vi "massajVoltageSimple.vi"() -> ()   [LabVIEW 2021]
uses:
  PicoMoLV/Global Variablesyes.vi
  C:/Program Files/New Focus/New Focus Picomotor Application/Samples/LabVIEW/Model 8742/LabVIEW 2009/CmdLib.dll
panel:
  out "Message":string
  in  "SetZero":bool
  in  "Set Velocity":dbl(slide)=10.0 min=10.0 max=4000.0 step=10.0 scale=0.0..2500.0
  out "FContact":bool caption="END CONTACT"
  in  "Volt Stop F":bool
  in  "Tab Control":enum32{"Coupler", "Feelers"}(tab)
  in  "Coupler On":bool
  out "Volt Plot C":dynamicdata(graph)
  out "Volt Plot F":dynamicdata(graph)
  in  "Feelers On":bool
  in  "Couple B":bool
  out "Direction":dbl
  in  "RIGHT":bool
  in  "LEFT":bool
  in  "Decouple":bool
  in  "LEFT/RIGHT COUPLE":bool
  out "CContact":bool caption="IN CONTACT"
  in  "Volt Stop C":bool
  in  "STOP LOOP 2":bool
  in  "Stop":bool
  out "error out":errorcluster
  out "In Motion":bool
  out "Status:":string
  out "Current Position:":string
  in  "Go":bool
  in  "Relative Move:":string
  in  "Selected Motor:":string(combo)
  in  "Selected Controller:":string(combo)
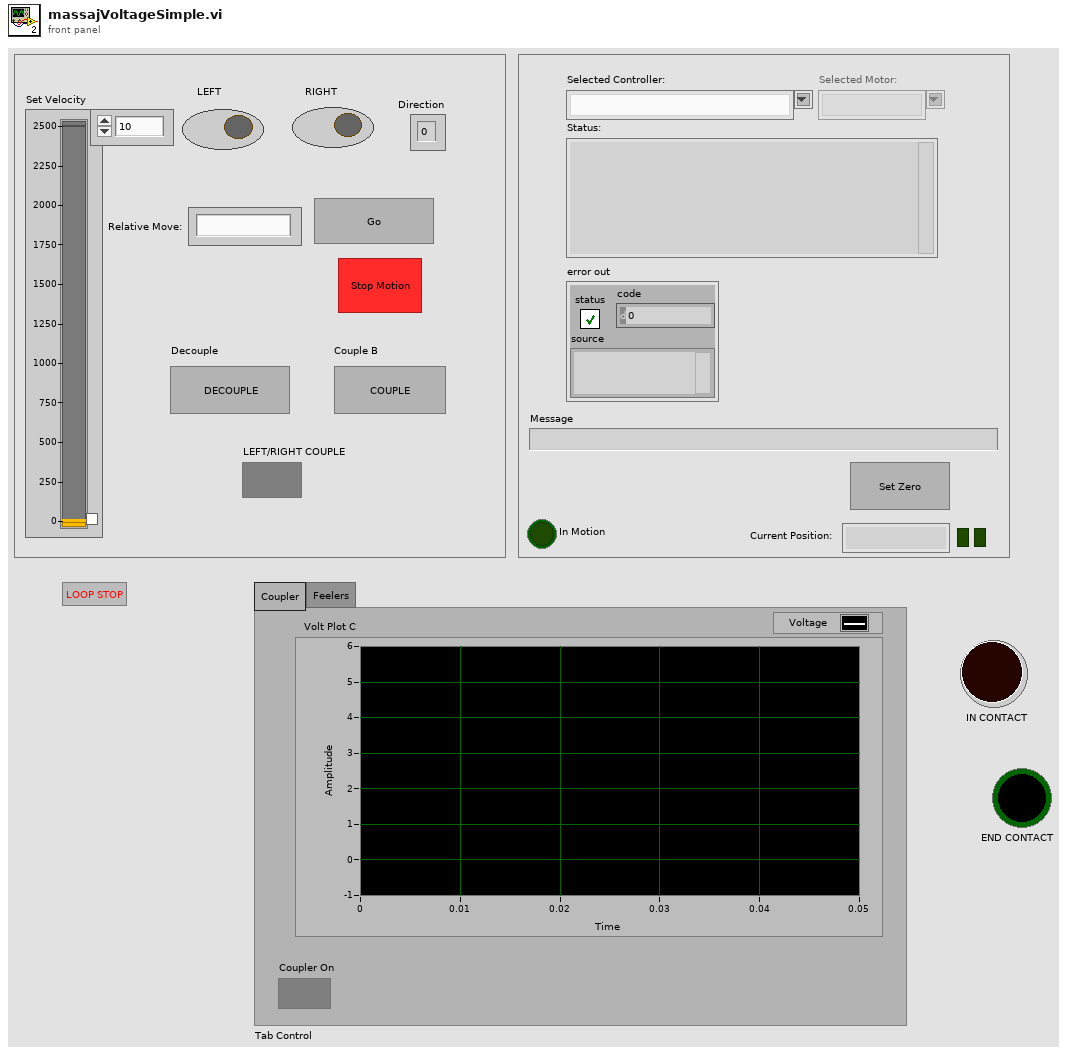
[diagram p1: front panel]
types:
  T1 = cluster{"Selected Controller:":refnum<vi>, "Selected Motor:":refnum<vi>, "Relative Move:":refnum<vi>, "Current Position:":refnum<vi>, "Go":refnum<vi>, "Stop":refnum<vi>}
  T2 = cluster{"DeviceKey":string, "Device Address":i32, "Controller Name":string}[]
  T3 = cluster{"DeviceKey":string, "Device Address":i32, "Controller Name":string}
  T4 = enum8{"Enabled", "Disabled", "Disabled and Grayed Out"}
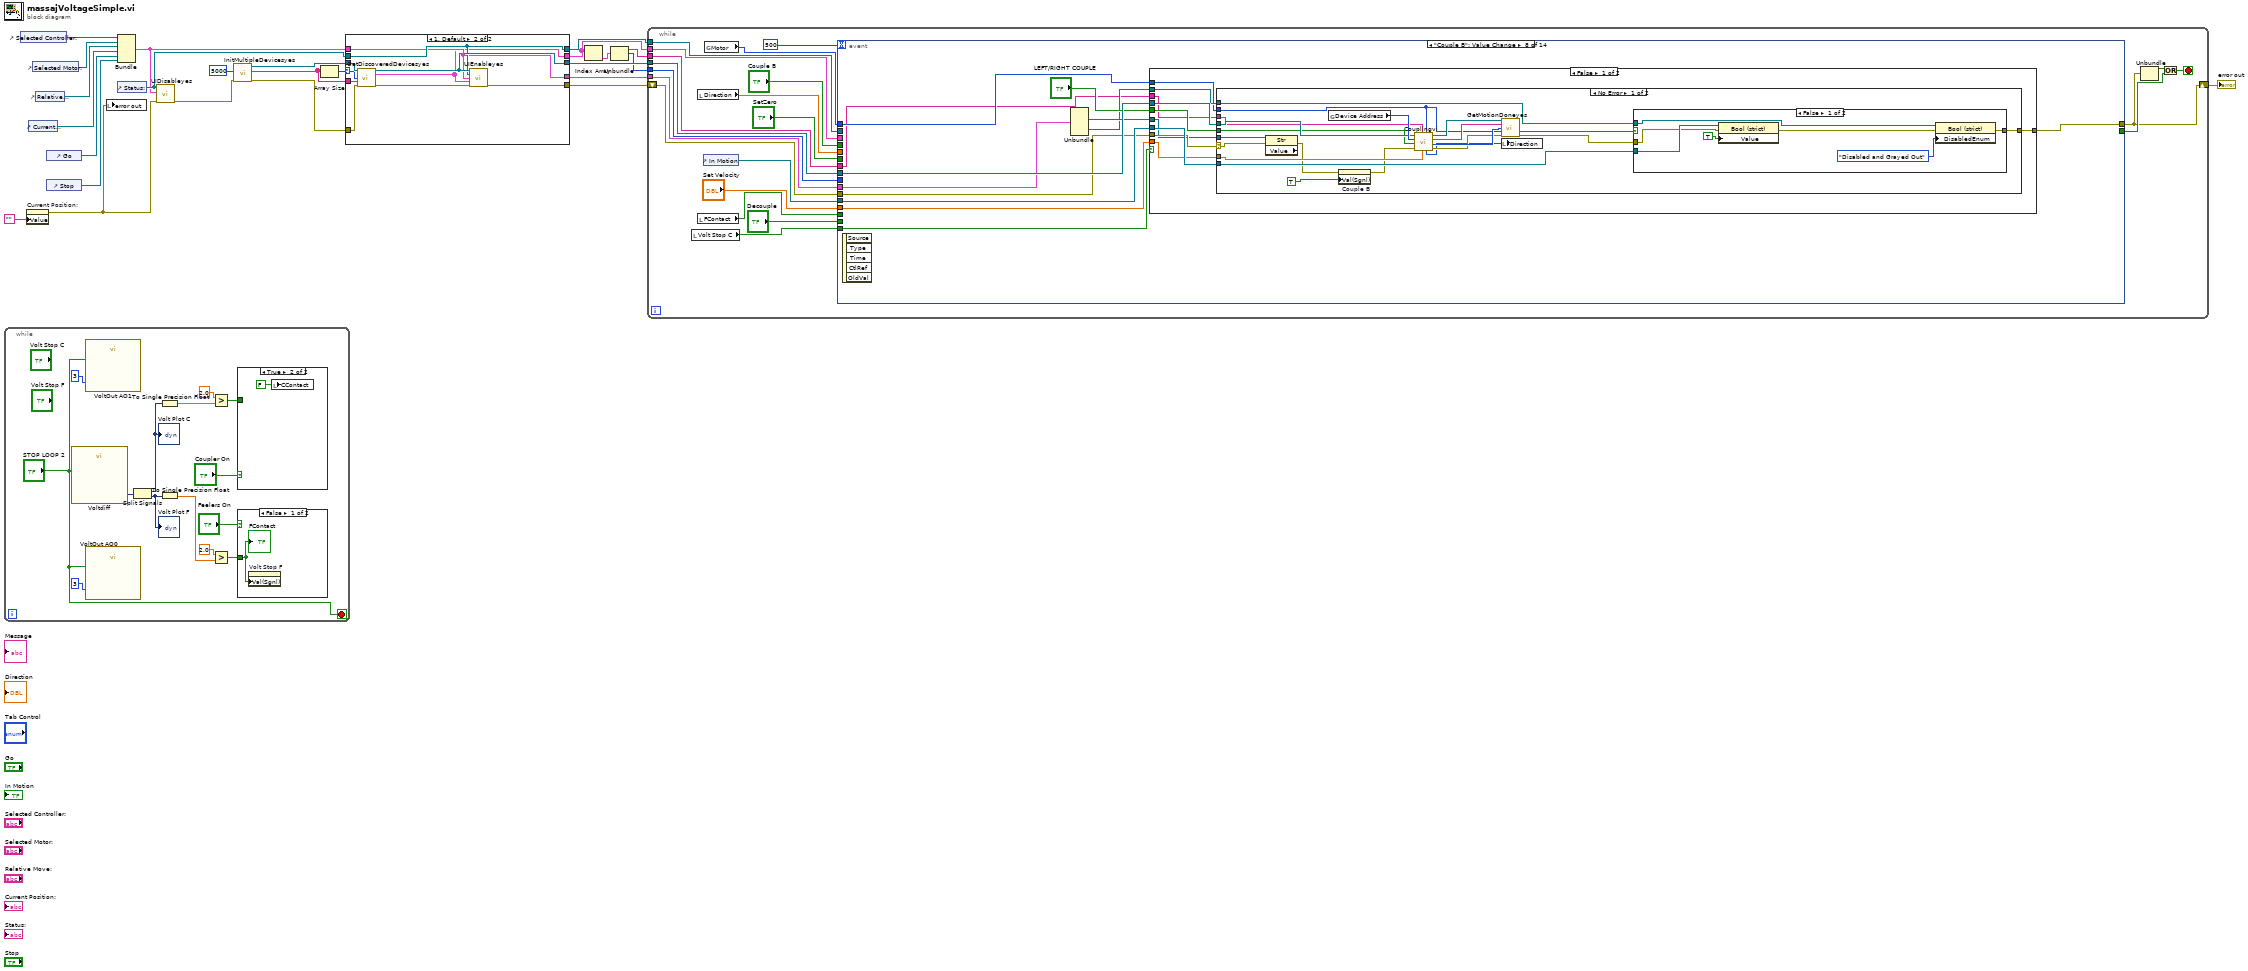
[diagram p0: block diagram]
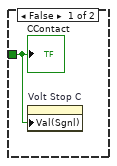
[diagram p2: hidden frame]
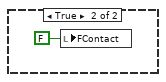
[diagram p3: hidden frame]
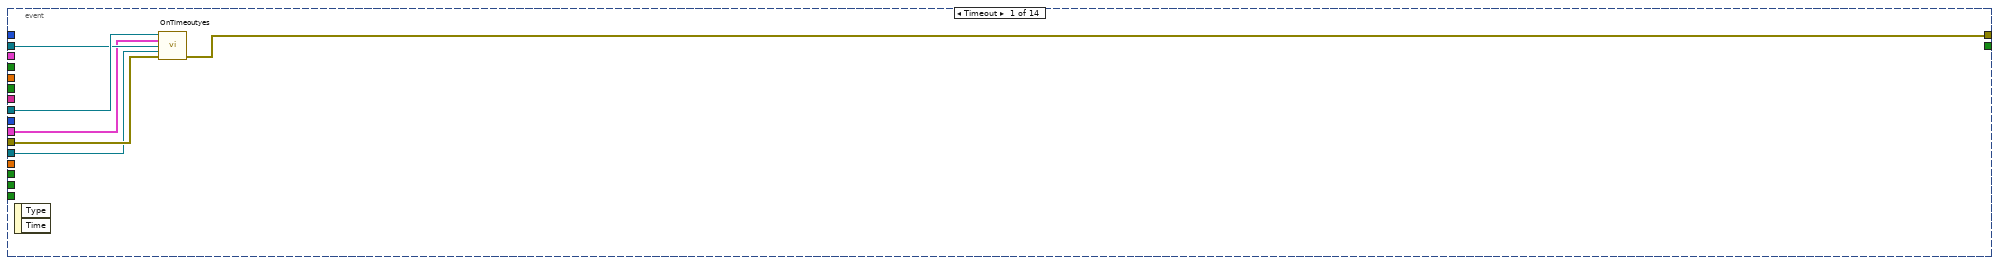
[diagram p4: hidden frame]
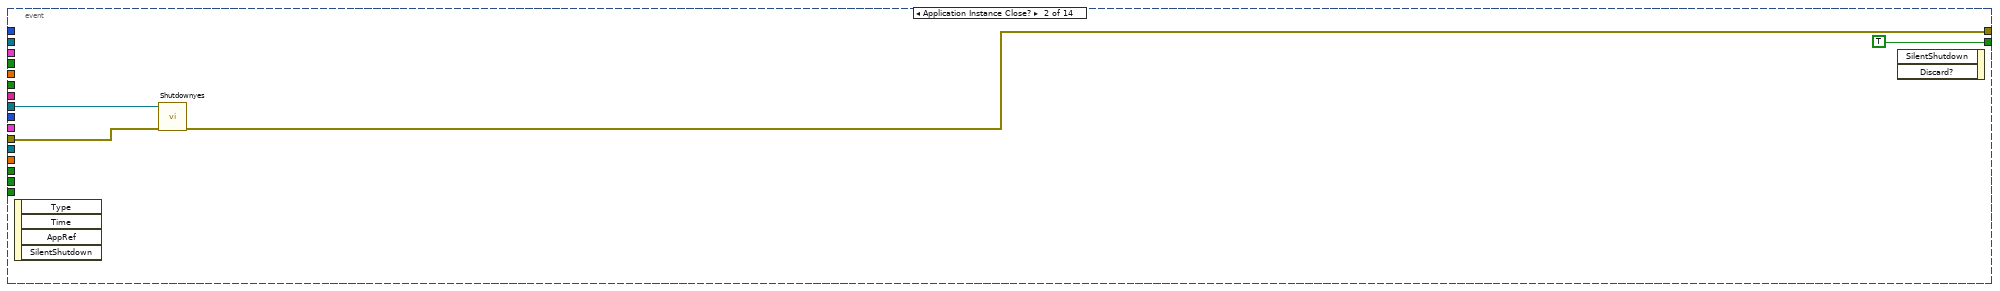
[diagram p5: hidden frame]
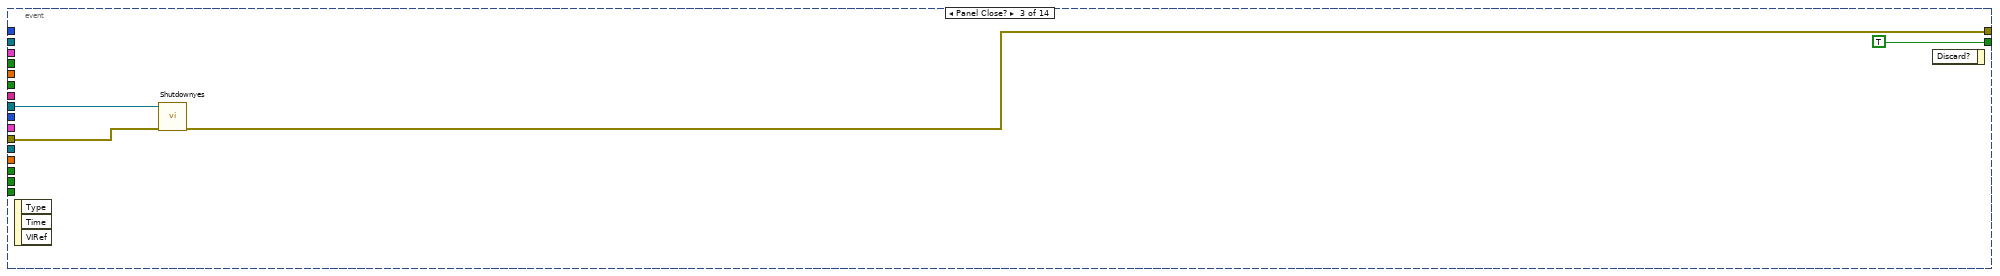
[diagram p6: hidden frame]
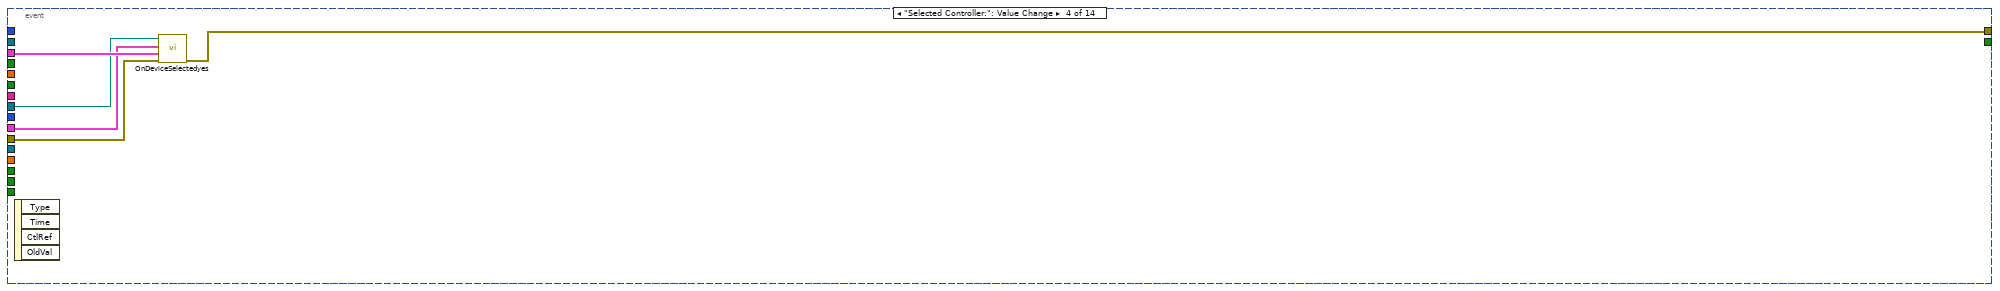
[diagram p7: hidden frame]
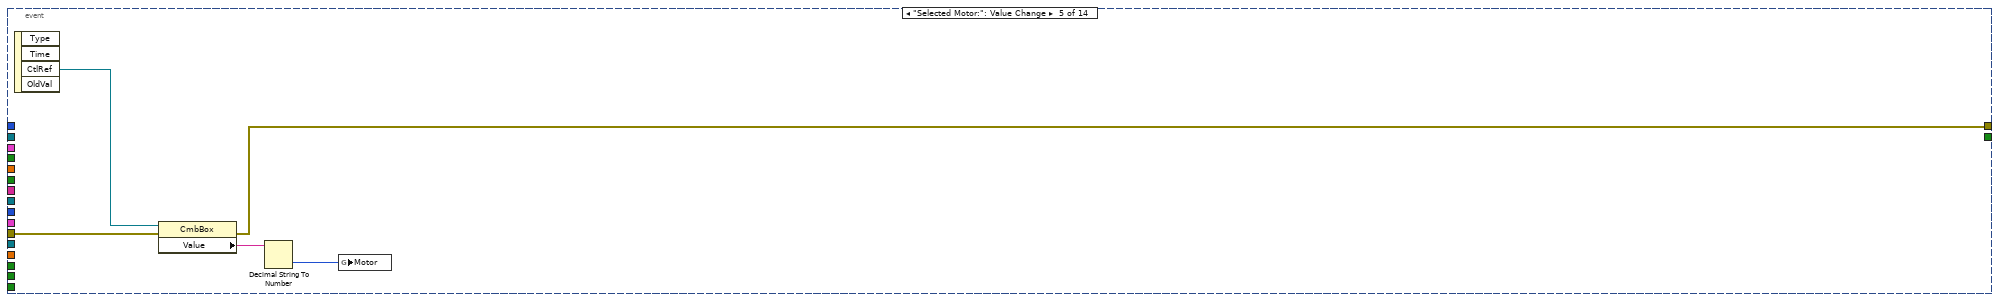
[diagram p8: hidden frame]
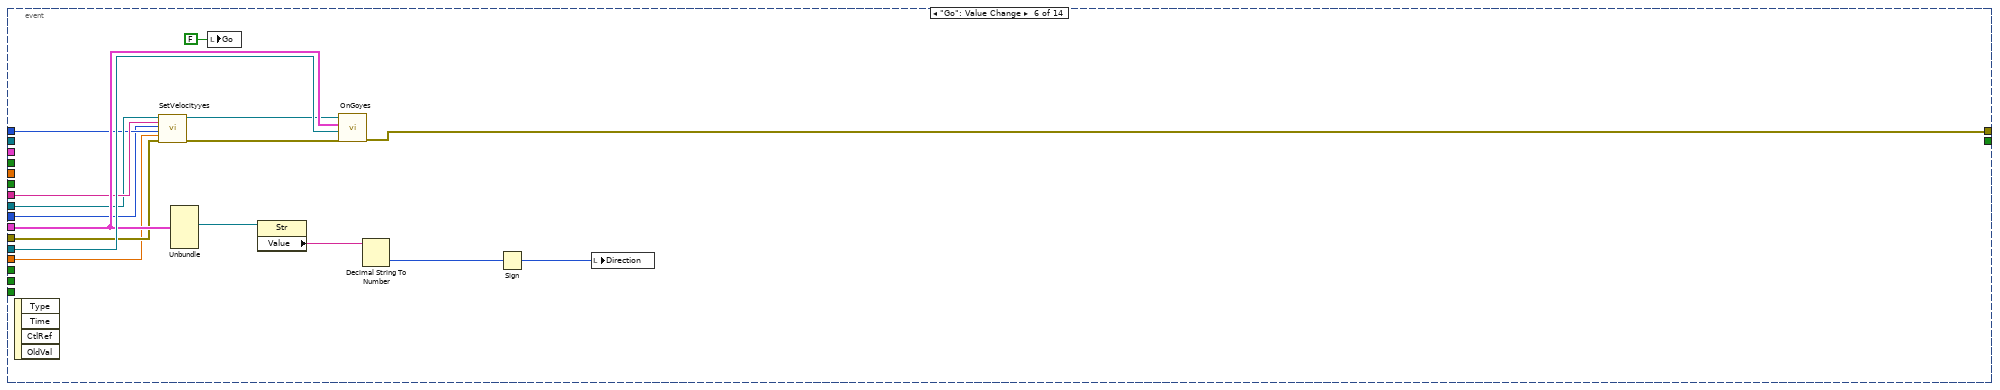
[diagram p9: hidden frame]
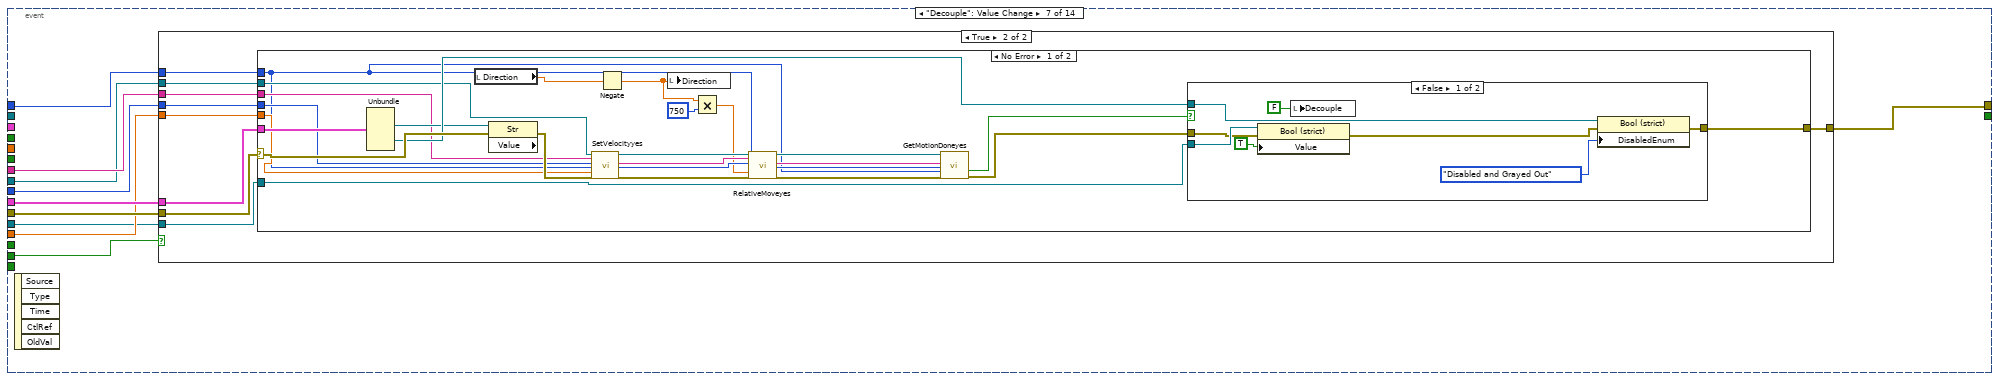
[diagram p10: hidden frame]
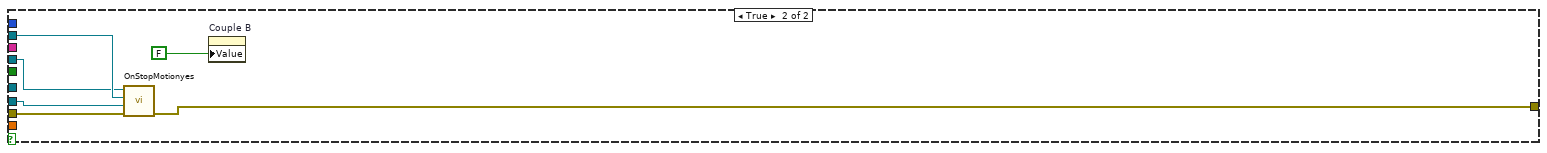
[diagram p16: hidden frame]
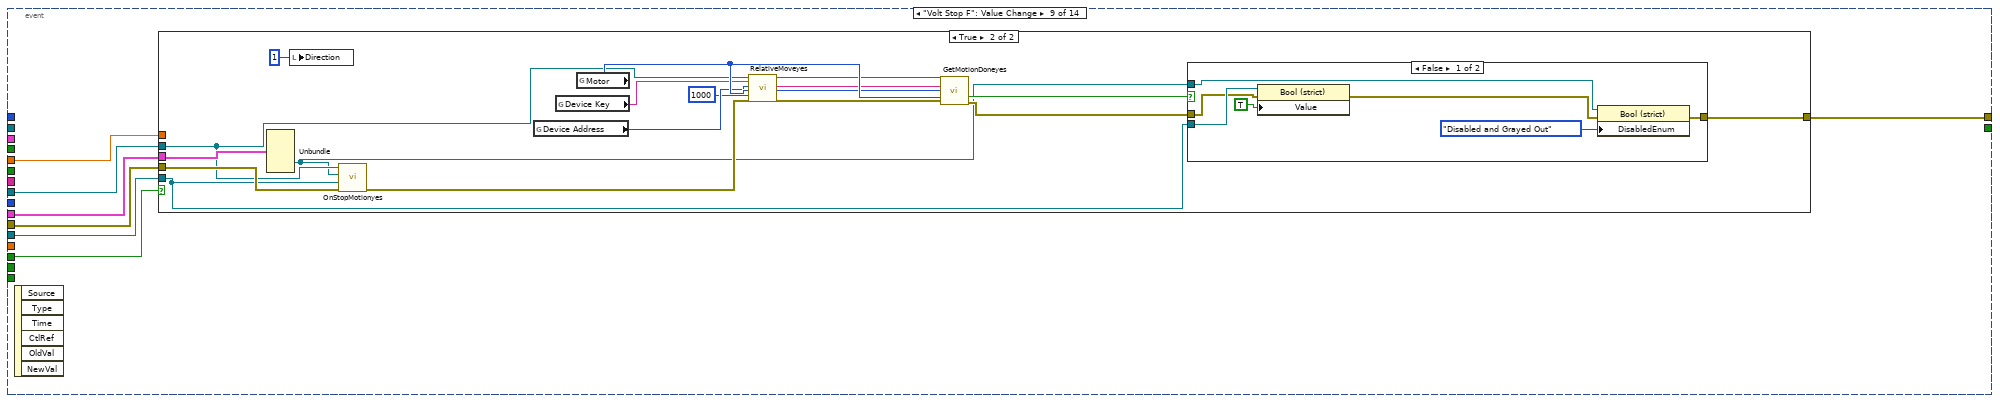
[diagram p17: hidden frame]
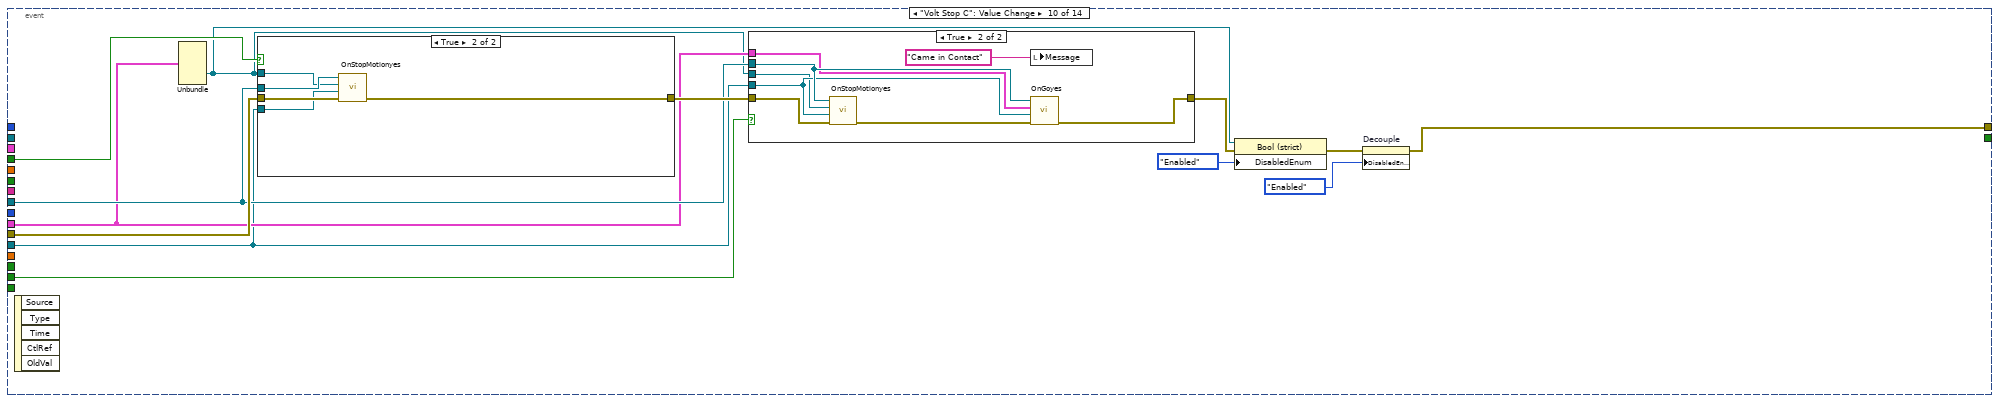
[diagram p20: hidden frame]
diagram:
  n1 = while {
    stop <- "STOP LOOP 2" stop-if-true
    n2 = call "Voltdiff"("stop (F)"="STOP LOOP 2") -> ("data"=w33:dynamicdata)  [unwired: 15 in, 3 out]
    n3 = call "VoltOut AO1"("data"=3, "stop (T)"="STOP LOOP 2") -> ()  [unwired: 16 in, 2 out]
    n4 = call "VoltOut AO0"("data"=3, "stop (T)"="STOP LOOP 2") -> ()  [unwired: 16 in, 2 out]
    n5 = Split Signals(w33) -> (w32:dynamicdata, w28:dynamicdata)  [unwired: 2 in]
    "Volt Plot C" <- w32
    "Volt Plot F" <- w28
    n6 = To Single Precision Float(number=w32) -> (single precision float=w37:sgl)
    n7 = To Single Precision Float(number=w28) -> (single precision float=w30:sgl)
    n8 = Greater?(x=2.0, y=w37) -> (0:w36:bool)
    n9 = Greater?(x=2.0, y=w30) -> (0:w29:bool)
    n10 = case shown="True" "Coupler On" {
      tunnel: w36 -> [w40 _]
      frame False {
        n11 = property on="Volt Stop C" class="Bool (strict)"("Val(Sgnl)"=w40) -> ()  [unwired: 2 in, 2 out]
        "CContact" <- w40
      }
      frame True {
        n12 = local write "CContact"(FALSE) -> ()
      }
    }
    n13 = case shown="False" "Feelers On" {
      tunnel: w29 -> [w42 _]
      frame False {
        n14 = property on="Volt Stop F" class="Bool (strict)"("Val(Sgnl)"=w42) -> ()  [unwired: 2 in, 2 out]
        "FContact" <- w42
      }
      frame True {
        n15 = local write "FContact"(FALSE) -> ()
      }
    }
  }
  n16 = control-ref of="Selected Controller:"() -> (w17:refnum<vi>)
  n17 = property on="Current Position:" class="Str"("Value"="") -> (error out=w8:errorcluster)  [unwired: 2 in, 1 out]
  n18 = control-ref of="Current Position:"() -> (w10:refnum<vi>)
  n19 = control-ref of="Selected Motor:"() -> (w25:refnum<vi>)
  n20 = control-ref of="Relative Move:"() -> (w24:refnum<vi>)
  n21 = control-ref of="Go"() -> (w6:refnum<vi>)
  n22 = control-ref of="Stop"() -> (w7:refnum<vi>)
  n23 = local write "error out"(w8) -> ()
  n24 = Bundle("Selected Controller:"=w17, "Selected Motor:"=w25, "Relative Move:"=w24, "Current Position:"=w10, "Go"=w6, "Stop"=w7) -> (w12:T1)  [unwired: 1 in]
  n25 = control-ref of="Status:"() -> (w16:refnum<vi>)
  n26 = call "UIDisableyes.vi"("error in (no error)"=w8, "UI"=w12, "Status:"=w16) -> ("error out"=w23:errorcluster)  [unwired: 8 in]
  n27 = call "InitMultipleDevicesyes.vi"("error in (no error)"=w23, "msecDelayForDiscovery"=5000) -> ("error out"=w20:errorcluster, "DeviceKey List Out"=w18:string[], "CmdLib Out"=w19:refnum<k24>)  [unwired: 3 in]
  n28 = Array Size(array=w18) -> (size(s)=w21:i32)
  n29 = case shown="1, Default" w21 {
    selector: w21 -> [_ w56]
    tunnel: w16 -> [w45 w53]
    tunnel: w20 -> [w49 w59]
    tunnel: w19 -> [w47 w60]
    tunnel: w18 -> [_ w58]
    tunnel: [w48 w55] -> w15
    tunnel: [w47 w54] -> w14
    tunnel: w12 -> [w46 w52]
    tunnel: [w46 w52] -> w11
    tunnel: [T2 [] ("Device Array") w51] -> w1
    tunnel: [w45 w53] -> w9
    frame 0 {
      n30 = call "AppendToOutputyes.vi"("error in"=w49, "Input String"="No devices were discovered.", "Output Refnum In"=w45) -> ("error out"=w48:errorcluster)  [unwired: 1 in, 1 out]
    }
    frame 1, Default {
      n31 = call "GetDiscoveredDevicesyes.vi"("CmdLib In"=w60, "Master Count"=w56, "DeviceKey List"=w58, "error in"=w59) -> ("CmdLib Out"=w54:refnum<k24>, "Device Array"=w51:T2, "error out"=w57:errorcluster)  [unwired: 9 in]
      n32 = call "UIEnableyes.vi"("CmdLib In"=w54, "Status:"=w53, "UI"=w52, "Device Array"=w51, "error in"=w57) -> ("error out"=w55:errorcluster)  [unwired: 10 in]
    }
  }
  n33 = Index Array(array=w1) -> (element=w4:T3)  [unwired: 1 in]
  n34 = Unbundle(w4) -> ("DeviceKey"=w3:string, "Device Address"=w2:i32)  [unwired: 1 out]
  n35 = while {
    tunnel: w14 -> [w80]
    tunnel: w11 -> [w79]
    tunnel: w1 -> [w78]
    shift-right: [w72] -> w5
    shift-left: w15 -> [w81]
    tunnel: w9 -> [w76]
    tunnel: w3 -> [w64]
    tunnel: w2 -> [w63]
    stop <- w71 stop-if-true
    n36 = local read "Volt Stop C"() -> (w68:bool)
    n37 = local read "Direction"() -> (w66:dbl)
    n38 = local read "FContact"() -> (w67:bool)
    n39 = control-ref of="In Motion"() -> (w73:refnum<vi>)
    n40 = global read "Global Variablesyes.vi" "Motor"() -> (w62:i32)
    n41 = event shown="[7] \"Couple B\": Value Change" {
      selector: _ -> [_ _ _ _ _ _ _ _ _ _ _ _ _ _]
      dyn-events: _ -> [_ _ _ _ _ _ _ _ _ _ _ _ _ _]
      timeout: 500 -> [_ _ _ _ _ _ _ _ _ _ _ _ _ _]
      tunnel: w81 -> [w87 w91 w94 w100 w103 w113 w128 w187 w239 w281 w302 w316 w363 w411]
      tunnel: w80 -> [w84 w90 w95 w97 _ w110 w122 w189 w240 w278 w298 w307 w360 w413]
      tunnel: [_ TRUE TRUE _ _ _ _ _ _ _ _ _ _ _] -> w74
      tunnel: [w86 w88 w92 w99 w102 w119 w131 w186 w238 w270 w301 w317 w366 w408] -> w72
      tunnel: w79 -> [w82 _ _ w96 _ w118 w129 w183 w241 w277 w300 w319 w367 _]
      tunnel: w78 -> [_ _ _ w98 _ _ _ _ _ _ _ _ _ _]
      tunnel: w76 -> [w83 _ _ _ _ _ _ _ _ _ _ _ _ _]
      tunnel: w73 -> [w85 _ _ _ _ w121 w126 w188 w237 w276 w303 w305 w357 _]
      tunnel: "Decouple" -> [_ _ _ _ _ _ w130 _ _ w275 _ _ _ _]
      tunnel: w68 -> [_ _ _ _ _ _ _ w179 _ _ _ _ _ _]
      tunnel: "Couple B" -> [_ _ _ _ _ _ _ _ _ w280 _ _ _ _]
      tunnel: w67 -> [_ _ _ _ _ _ _ _ w242 _ _ _ _ _]
      tunnel: w66 -> [_ _ _ _ _ _ _ _ w236 _ _ _ _ _]
      tunnel: "Set Velocity" -> [_ _ _ _ _ w108 w127 w181 _ _ _ w310 w364 _]
      tunnel: w64 -> [_ _ _ _ _ w111 w123 w178 _ _ _ w309 w361 w412]
      tunnel: w63 -> [_ _ _ _ _ w106 w125 _ _ _ _ w308 w362 w409]
      tunnel: w62 -> [_ _ _ _ _ w107 w124 w180 _ _ _ w306 w359 w410]
      tunnel: "SetZero" -> [_ _ _ _ _ _ _ _ _ _ _ _ _ w414]
      event Timeout {
        n42 = event-data() -> ()  [unwired: 1 in, 2 out]
        n43 = call "OnTimeoutyes.vi"("CmdLib In"=w84, "UI"=w82, "Status:"=w83, "In Motion"=w85, "error in"=w87) -> ("error out"=w86:errorcluster)  [unwired: 10 in]
      }
      event Application Instance Close? {
        n44 = event-data() -> ()  [unwired: 1 in, 4 out]
        n45 = call "Shutdownyes.vi"("error in (no error)"=w91, "CmdLib In"=w90) -> ("error out"=w88:errorcluster)  [unwired: 4 in, 1 out]
        n46 = event-data() -> ()  [unwired: 3 in, 1 out]
      }
      event Panel Close? {
        n47 = event-data() -> ()  [unwired: 1 in, 3 out]
        n48 = call "Shutdownyes.vi"("error in (no error)"=w94, "CmdLib In"=w95) -> ("error out"=w92:errorcluster)  [unwired: 4 in, 1 out]
        n49 = event-data() -> ()  [unwired: 2 in, 1 out]
      }
      event "Selected Controller:": Value Change {
        n50 = event-data() -> ()  [unwired: 1 in, 4 out]
        n51 = call "OnDeviceSelectedyes.vi"("error in"=w100, "Device Array"=w98, "UI"=w96, "CmdLib In"=w97) -> ("error out"=w99:errorcluster)  [unwired: 7 in]
      }
      event "Selected Motor:": Value Change {
        n52 = event-data() -> ("CtlRef"=w101:refnum<vi>)  [unwired: 1 in, 3 out]
        n53 = property class="CmbBox"(reference=w101, error in=w103) -> (error out=w102:errorcluster, "Value"=w105:string)  [unwired: 1 out]
        n54 = Decimal String To Number(string=w105) -> (number=w104:i32)  [unwired: 2 in, 1 out]
        n55 = global write "Global Variablesyes.vi" "Motor"(w104) -> ()
      }
      event "Go": Value Change {
        n56 = event-data() -> ()  [unwired: 1 in, 4 out]
        n57 = call "SetVelocityyes.vi"("CmdLib In"=w110, "DeviceKey In"=w111, "Device Address In"=w106, "Motor"=w107, "Steps Per Sec"=w108, "error in (no error)"=w113) -> ("CmdLib Out"=w109:refnum<k24>, "error out"=w112:errorcluster)  [unwired: 10 in, 2 out]
        n58 = Unbundle(w118) -> ("Relative Move:"=w116:refnum<vi>)  [unwired: 5 out]
        n59 = local write "Go"(FALSE ("Go")) -> ()
        n60 = property class="Str"(reference=w116) -> ("Value"=w117:string)  [unwired: 1 in, 2 out]
        n61 = call "OnGoyes.vi"("error in"=w112, "In Motion"=w121, "UI"=w118, "CmdLib Out"=w109) -> ("error out"=w119:errorcluster)  [unwired: 7 in]
        n62 = Decimal String To Number(string=w117) -> (number=w115:i32)  [unwired: 2 in, 1 out]
        n63 = Sign(1:w115) -> (0:w114:i32)
        n64 = local write "Direction"(w114) -> ()
      }
      event "Decouple": Value Change {
        n65 = event-data() -> ()  [unwired: 1 in, 5 out]
        n66 = case shown="True" w130 {
          tunnel: w129 -> [_ w141]
          tunnel: w122 -> [_ w140]
          tunnel: w126 -> [_ w139]
          tunnel: w128 -> [w132 w138]
          tunnel: [w132 w137] -> w131
          tunnel: w123 -> [_ w136]
          tunnel: w125 -> [_ w135]
          tunnel: w124 -> [_ w134]
          tunnel: w127 -> [_ w133]
          frame False {
          }
          frame True {
            n67 = case shown="No Error" w138 {
              selector: w138 -> [w164 w177]
              tunnel: [w165 w177] -> w137
              tunnel: w141 -> [w161 _]
              tunnel: w140 -> [w155 _]
              tunnel: w139 -> [w160 _]
              tunnel: w136 -> [w152 _]
              tunnel: w135 -> [w151 _]
              tunnel: w134 -> [w145 _]
              tunnel: w133 -> [w146 _]
              frame No Error {
                n68 = Unbundle(w161) -> ("Relative Move:"=w162:refnum<vi>, "Go"=w163:refnum<vi>)  [unwired: 4 out]
                n69 = local read "Direction"() -> (w159:dbl)
                n70 = property class="Str" props=["Value"](reference=w162, error in=w164) -> (error out=w158:errorcluster)  [unwired: 2 out]
                n71 = call "SetVelocityyes.vi"("CmdLib In"=w155, "DeviceKey In"=w152, "Device Address In"=w151, "Motor"=w145, "Steps Per Sec"=w146, "error in (no error)"=w158) -> ("CmdLib Out"=w154:refnum<k24>, "DeviceKey Out"=w150:string, "Device Address Out"=w148:i32, "error out"=w157:errorcluster)  [unwired: 10 in]
                n72 = Negate(x=w159) -> (-x=w143:dbl)
                n73 = local write "Direction"(w143) -> ()
                n74 = Multiply(x=w143, y=750) -> (x*y=w142:dbl)
                n75 = call "RelativeMoveyes.vi"("CmdLib In"=w154, "DeviceKey In"=w150, "Device Address In"=w148, "Motor"=w145, "Relative Steps"=w142, "error in (no error)"=w157) -> ("CmdLib Out"=w153:refnum<k24>, "DeviceKey Out"=w149:string, "Device Address Out"=w147:i32, "error out"=w156:errorcluster)  [unwired: 10 in]
                n76 = call "GetMotionDoneyes.vi"("CmdLib In"=w153, "DeviceKey In"=w149, "Device Address In"=w147, "Motor"=w145, "error in (no error)"=w156) -> ("Is Motion Done"=w167:bool, "error out"=w166:errorcluster)  [unwired: 6 in, 3 out]
                n77 = case shown="False" w167 {
                  tunnel: [w169 w176] -> w165
                  tunnel: w163 -> [w174 _]
                  tunnel: w166 -> [w171 w176]
                  tunnel: w160 -> [w173 _]
                  frame False {
                    n78 = property class="Bool (strict)"(reference=w173, error in=w171, "Value"=TRUE) -> (error out=w170:errorcluster)  [unwired: 1 out]
                    n79 = local write "Decouple"(FALSE) -> ()
                    n80 = property class="Bool (strict)"(reference=w174, error in=w170, "DisabledEnum"=T4."Disabled and Grayed Out" ("Disabled")) -> (error out=w169:errorcluster)  [unwired: 1 out]
                  }
                  frame True {
                  }
                }
              }
              frame Error {
              }
            }
          }
        }
      }
      event "Couple B": Value Change {
        n81 = event-data() -> ()  [unwired: 1 in, 5 out]
        n82 = Unbundle(w183) -> ("Relative Move:"=w184:refnum<vi>, "Go"=w182:refnum<vi>)  [unwired: 4 out]
        n83 = case shown="False" w179 {
          tunnel: w189 -> [w199 w232]
          tunnel: w188 -> [w198 w231]
          tunnel: w187 -> [w197 w235]
          tunnel: [w196 w234] -> w186
          tunnel: "LEFT/RIGHT COUPLE" -> [w195 _]
          tunnel: w184 -> [w194 _]
          tunnel: w182 -> [w193 w233]
          tunnel: w181 -> [w192 _]
          tunnel: w180 -> [w191 _]
          tunnel: w178 -> [w190 _]
          frame False {
            n84 = case shown="No Error" w197 {
              selector: w197 -> [w212 w229]
              tunnel: [w214 w229] -> w196
              tunnel: w199 -> [w211 _]
              tunnel: w198 -> [w210 _]
              tunnel: w195 -> [w209 _]
              tunnel: w194 -> [w207 _]
              tunnel: w193 -> [w206 _]
              tunnel: w192 -> [w205 _]
              tunnel: w191 -> [w204 _]
              tunnel: w190 -> [w203 _]
              frame No Error {
                n85 = property class="Str" props=["Value"](reference=w207, error in=w212) -> (error out=w202:errorcluster)  [unwired: 2 out]
                n86 = global read "Global Variablesyes.vi" "Device Address"() -> (w213:i32)
                n87 = property on="Couple B" class="Bool (strict)"(error in=w202, "Val(Sgnl)"=TRUE) -> (error out=w201:errorcluster)  [unwired: 1 in, 1 out]
                n88 = call "Couplingvi.vi"("Motor"=w204, "Step per Sec"=w205, "Device Key"=w203, "error in (no error)"=w201, "LEFT/RIGHT COUPLE"=w209, "Device Address"=w213, ".NET Refnum in"=w211) -> ("error out"=w215:errorcluster, "Device Address Out"=w219:i32, "DeviceKey Out"=w218:string, ".NET Refnum out"=w217:refnum<k24>, "Direction"=w208:i32)
                n89 = call "GetMotionDoneyes.vi"("CmdLib In"=w217, "DeviceKey In"=w218, "Device Address In"=w219, "Motor"=w204, "error in (no error)"=w215) -> ("Is Motion Done"=w220:bool, "error out"=w216:errorcluster)  [unwired: 6 in, 3 out]
                n90 = local write "Direction"(w208) -> ()
                n91 = case shown="False" w220 {
                  tunnel: [w221 w228] -> w214
                  tunnel: w206 -> [w226 _]
                  tunnel: w216 -> [w223 w228]
                  tunnel: w210 -> [w225 _]
                  frame False {
                    n92 = property class="Bool (strict)"(reference=w225, error in=w223, "Value"=TRUE) -> (error out=w222:errorcluster)  [unwired: 1 out]
                    n93 = property class="Bool (strict)"(reference=w226, error in=w222, "DisabledEnum"=T4."Disabled and Grayed Out" ("Disabled")) -> (error out=w221:errorcluster)  [unwired: 1 out]
                  }
                  frame True {
                  }
                }
              }
              frame Error {
              }
            }
          }
          frame True {
            n94 = call "OnStopMotionyes.vi"("error in"=w235, "In Motion"=w231, "Go"=w233, "CmdLib In"=w232) -> ("error out"=w234:errorcluster)  [unwired: 7 in]
            n95 = property on="Couple B" class="Bool (strict)"("Value"=FALSE) -> ()  [unwired: 2 in, 2 out]
          }
        }
      }
      event "Volt Stop F": Value Change {
        n96 = event-data() -> ()  [unwired: 1 in, 6 out]
        n97 = case shown="True" w242 {
          tunnel: w241 -> [_ w261]
          tunnel: w240 -> [_ w247]
          tunnel: w239 -> [w243 w260]
          tunnel: [w243 w245] -> w238
          tunnel: w237 -> [_ w248]
          tunnel: w236 -> [_ _]
          frame False {
          }
          frame True {
            n98 = Unbundle(w261) -> ("Go"=w246:refnum<vi>)  [unwired: 5 out]
            n99 = local write "Direction"(1) -> ()
            n100 = call "OnStopMotionyes.vi"("error in"=w260, "In Motion"=w248, "Go"=w246, "CmdLib In"=w247) -> ("error out"=w249:errorcluster)  [unwired: 7 in]
            n101 = global read "Global Variablesyes.vi" "Device Address"() -> (w252:i32)
            n102 = global read "Global Variablesyes.vi" "Device Key"() -> (w251:string)
            n103 = global read "Global Variablesyes.vi" "Motor"() -> (w258:i32)
            n104 = call "RelativeMoveyes.vi"("CmdLib In"=w247, "DeviceKey In"=w251, "Device Address In"=w252, "Motor"=w258, "Relative Steps"=1000, "error in (no error)"=w249) -> ("CmdLib Out"=w255:refnum<k24>, "DeviceKey Out"=w256:string, "Device Address Out"=w257:i32, "error out"=w253:errorcluster)  [unwired: 10 in]
            n105 = call "GetMotionDoneyes.vi"("CmdLib In"=w255, "DeviceKey In"=w256, "Device Address In"=w257, "Motor"=w258, "error in (no error)"=w253) -> ("Is Motion Done"=w259:bool, "error out"=w254:errorcluster)  [unwired: 6 in, 3 out]
            n106 = case shown="False" w259 {
              tunnel: [w262 w269] -> w245
              tunnel: w246 -> [w267 _]
              tunnel: w254 -> [w264 w269]
              tunnel: w248 -> [w266 _]
              frame False {
                n107 = property class="Bool (strict)"(reference=w266, error in=w264, "Value"=TRUE) -> (error out=w263:errorcluster)  [unwired: 1 out]
                n108 = property class="Bool (strict)"(reference=w267, error in=w263, "DisabledEnum"=T4."Disabled and Grayed Out" ("Disabled")) -> (error out=w262:errorcluster)  [unwired: 1 out]
              }
              frame True {
              }
            }
          }
        }
      }
      event "Volt Stop C": Value Change {
        n109 = event-data() -> ()  [unwired: 1 in, 5 out]
        n110 = Unbundle(w277) -> ("Go"=w274:refnum<vi>)  [unwired: 5 out]
        n111 = case shown="True" w280 {
          tunnel: w281 -> [w292 w297]
          tunnel: w278 -> [_ w295]
          tunnel: w274 -> [_ w294]
          tunnel: [w292 w296] -> w279
          tunnel: w276 -> [_ w293]
          frame False {
          }
          frame True {
            n112 = call "OnStopMotionyes.vi"("error in"=w297, "In Motion"=w293, "Go"=w294, "CmdLib In"=w295) -> ("error out"=w296:errorcluster)  [unwired: 7 in]
          }
        }
        n113 = case shown="True" w275 {
          tunnel: w279 -> [w283 w291]
          tunnel: [w283 w289] -> w273
          tunnel: w278 -> [_ w288]
          tunnel: w277 -> [_ w287]
          tunnel: w276 -> [_ w286]
          tunnel: w274 -> [_ w285]
          frame False {
          }
          frame True {
            n114 = call "OnStopMotionyes.vi"("error in"=w291, "In Motion"=w286, "Go"=w285, "CmdLib In"=w288) -> ("error out"=w290:errorcluster)  [unwired: 7 in]
            n115 = local write "Message"("Came in Contact") -> ()
            n116 = call "OnGoyes.vi"("error in"=w290, "In Motion"=w286, "UI"=w287, "CmdLib Out"=w288) -> ("error out"=w289:errorcluster)  [unwired: 7 in]
          }
        }
        n117 = property class="Bool (strict)"(reference=w274, error in=w273, "DisabledEnum"=T4."Enabled" ("Disabled")) -> (error out=w271:errorcluster)  [unwired: 1 out]
        n118 = property on="Decouple" class="Bool (strict)"(error in=w271, "DisabledEnum"=T4."Enabled" ("Disabled")) -> (error out=w270:errorcluster)  [unwired: 1 in, 1 out]
      }
      event "Stop": Value Change {
        n119 = event-data() -> ()  [unwired: 1 in, 5 out]
        n120 = Unbundle(w300) -> ("Go"=w299:refnum<vi>)  [unwired: 5 out]
        n121 = local write "Stop"(FALSE) -> ()
        n122 = call "OnStopMotionyes.vi"("error in"=w302, "In Motion"=w303, "Go"=w299, "CmdLib In"=w298) -> ("error out"=w301:errorcluster)  [unwired: 7 in]
      }
      event "LEFT": Value Change {
        n123 = event-data() -> ()  [unwired: 1 in, 6 out]
        n124 = call "SetVelocityyes.vi"("CmdLib In"=w307, "DeviceKey In"=w309, "Device Address In"=w308, "Motor"=w306, "Steps Per Sec"=w310, "error in (no error)"=w316) -> ("CmdLib Out"=w312:refnum<k24>, "DeviceKey Out"=w314:string, "Device Address Out"=w313:i32, "error out"=w315:errorcluster)  [unwired: 10 in]
        n125 = Unbundle(w319) -> ("Go"=w311:refnum<vi>)  [unwired: 5 out]
        n126 = case shown="True" "LEFT" {
          tunnel: w305 -> [w324 w332]
          tunnel: [w323 w331] -> w317
          tunnel: w311 -> [w322 w330]
          tunnel: w306 -> [_ w329]
          tunnel: w312 -> [w320 w328]
          tunnel: w314 -> [_ w327]
          tunnel: w313 -> [_ w326]
          tunnel: w315 -> [w321 w325]
          frame False {
            n127 = call "OnStopMotionyes.vi"("error in"=w321, "In Motion"=w324, "Go"=w322, "CmdLib In"=w320) -> ("error out"=w323:errorcluster)  [unwired: 7 in]
          }
          frame True {
            n128 = case shown="No Error" w325 {
              selector: w325 -> [w333 w356]
              tunnel: [w345 w356] -> w331
              tunnel: w332 -> [w344 _]
              tunnel: w330 -> [w343 _]
              tunnel: w329 -> [w337 _]
              tunnel: w328 -> [w336 _]
              tunnel: w327 -> [w335 _]
              tunnel: w326 -> [w334 _]
              frame No Error {
                (unwired) 1
                n129 = call "JogPositiveyes.vi"("CmdLib In"=w336, "DeviceKey In"=w335, "Device Address In"=w334, "Motor"=w337, "error in (no error)"=w333) -> ("CmdLib Out"=w341:refnum<k24>, "DeviceKey Out"=w340:string, "Device Address Out"=w339:i32, "error out"=w338:errorcluster)  [unwired: 7 in]
                n130 = local write "Direction"(1) -> ()
                n131 = call "GetMotionDoneyes.vi"("CmdLib In"=w341, "DeviceKey In"=w340, "Device Address In"=w339, "Motor"=w337, "error in (no error)"=w338) -> ("Is Motion Done"=w347:bool, "error out"=w346:errorcluster)  [unwired: 6 in, 3 out]
                n132 = case shown="False" w347 {
                  tunnel: [w348 w355] -> w345
                  tunnel: w343 -> [w353 _]
                  tunnel: w346 -> [w350 w355]
                  tunnel: w344 -> [w352 _]
                  frame False {
                    n133 = property class="Bool (strict)"(reference=w352, error in=w350, "Value"=TRUE) -> (error out=w349:errorcluster)  [unwired: 1 out]
                    n134 = property class="Bool (strict)"(reference=w353, error in=w349, "DisabledEnum"=T4."Disabled and Grayed Out" ("Disabled")) -> (error out=w348:errorcluster)  [unwired: 1 out]
                  }
                  frame True {
                  }
                }
              }
              frame Error {
              }
            }
          }
        }
      }
      event "RIGHT": Value Change {
        n135 = event-data() -> ()  [unwired: 1 in, 6 out]
        n136 = Unbundle(w367) -> ("Go"=w358:refnum<vi>)  [unwired: 5 out]
        n137 = case shown="True" "RIGHT" {
          tunnel: w360 -> [w372 w381]
          tunnel: w357 -> [w371 w380]
          tunnel: w363 -> [w370 w379]
          tunnel: [w369 w378] -> w366
          tunnel: w358 -> [w368 w377]
          tunnel: w362 -> [_ w376]
          tunnel: w361 -> [_ w375]
          tunnel: w359 -> [_ w374]
          tunnel: w364 -> [_ w373]
          frame False {
            n138 = call "OnStopMotionyes.vi"("error in"=w370, "In Motion"=w371, "Go"=w368, "CmdLib In"=w372) -> ("error out"=w369:errorcluster)  [unwired: 7 in]
          }
          frame True {
            n139 = case shown="No Error" w379 {
              selector: w379 -> [w391 w407]
              tunnel: [w392 w407] -> w378
              tunnel: w381 -> [w390 _]
              tunnel: w380 -> [w389 _]
              tunnel: w377 -> [w388 _]
              tunnel: w376 -> [w385 _]
              tunnel: w375 -> [w384 _]
              tunnel: w374 -> [w383 _]
              tunnel: w373 -> [w382 _]
              frame No Error {
                n140 = call "Couplingvi.vi"("Motor"=w383, "Step per Sec"=w382, "Device Key"=w384, "error in (no error)"=w391, "LEFT/RIGHT COUPLE"=FALSE, "Device Address"=w385, ".NET Refnum in"=w390) -> ("error out"=w393:errorcluster, "Device Address Out"=w397:i32, "DeviceKey Out"=w396:string, ".NET Refnum out"=w395:refnum<k24>, "Direction"=w386:i32)
                n141 = call "GetMotionDoneyes.vi"("CmdLib In"=w395, "DeviceKey In"=w396, "Device Address In"=w397, "Motor"=w383, "error in (no error)"=w393) -> ("Is Motion Done"=w398:bool, "error out"=w394:errorcluster)  [unwired: 6 in, 3 out]
                n142 = local write "Direction"(w386) -> ()
                n143 = case shown="False" w398 {
                  tunnel: [w399 w406] -> w392
                  tunnel: w388 -> [w404 _]
                  tunnel: w394 -> [w401 w406]
                  tunnel: w389 -> [w403 _]
                  frame False {
                    n144 = property class="Bool (strict)"(reference=w403, error in=w401, "Value"=TRUE) -> (error out=w400:errorcluster)  [unwired: 1 out]
                    n145 = property class="Bool (strict)"(reference=w404, error in=w400, "DisabledEnum"=T4."Disabled and Grayed Out" ("Disabled")) -> (error out=w399:errorcluster)  [unwired: 1 out]
                  }
                  frame True {
                  }
                }
              }
              frame Error {
              }
            }
          }
        }
      }
      event "SetZero": Value Change {
        n146 = event-data() -> ()  [unwired: 1 in, 6 out]
        n147 = case shown="True" w414 {
          tunnel: w411 -> [w415 w421]
          tunnel: w410 -> [_ w420]
          tunnel: w412 -> [_ w419]
          tunnel: w409 -> [_ w418]
          tunnel: [w415 w417] -> w408
          tunnel: w413 -> [_ w416]
          frame False {
          }
          frame True {
            n148 = case shown="No Error" w421 {
              selector: w421 -> [w427 w436]
              tunnel: w416 -> [w429 _]
              tunnel: w420 -> [w423 _]
              tunnel: w419 -> [w428 _]
              tunnel: [w424 w436] -> w417
              tunnel: w418 -> [w422 _]
              frame No Error {
                n149 = invoke class="CmdLib8742" method="SetZeroPosition"(reference=w429, error in=w427, "deviceKey"=w428, "deviceAddress"=w422, "motor"=w423) -> (error out=w425:errorcluster, "SetZeroPosition"=w426:bool)  [unwired: 1 in, 4 out]
                n150 = case shown="False" w426 {
                  tunnel: w425 -> [w434 w435]
                  tunnel: [w433 w435] -> w424
                  frame False {
                    n151 = Bundle By Name(cluster=w434, "status"=TRUE, "code"=1, "source"="SetZeroPosition.vi I/O Error.") -> (w433:errorcluster)
                  }
                  frame True {
                  }
                }
              }
              frame Error {
              }
            }
          }
        }
      }
    }
    n152 = Unbundle(w72) -> ("status"=w75:bool)  [unwired: 2 out]
    n153 = Or(x=w75, y=w74) -> (x .or. y?=w71:bool)
  }
  "error out" <- w5
